vi "Config.Simulate.Set.vi"(8 "error in (no error)":errorcluster, 9 "Simulate":bool, 11 "Config Folder":path=path "C:/DDCS/Config") -> (0 "error out":errorcluster)   [LabVIEW 2024, in "EQMF.lvlib" / "Config Utils.lvlib"]
doc: "This VI writes the simulate flag (Boolean) to the station config INI file (Local Station.ini).\nThe Simulate flag is stored in section \"Simulate\" item \"Enable\".\n\nINPUTS:\n<B>Config folder</B> - This is the folder where config files are stored.\n<B>Simulate</B> - This is the state to be stored. TRUE equals Simulate is ON.\n\nOUTPUTS:\nNone\n\nERRORS: \nIf the config file cannot be created or written to, an error will be reported."
uses:
  Config Utils.lvlib
  <vilib>/Utility/config.llb/Write Key (Boolean).vi
  <vilib>/Utility/config.llb/NI_LVConfig.lvlib
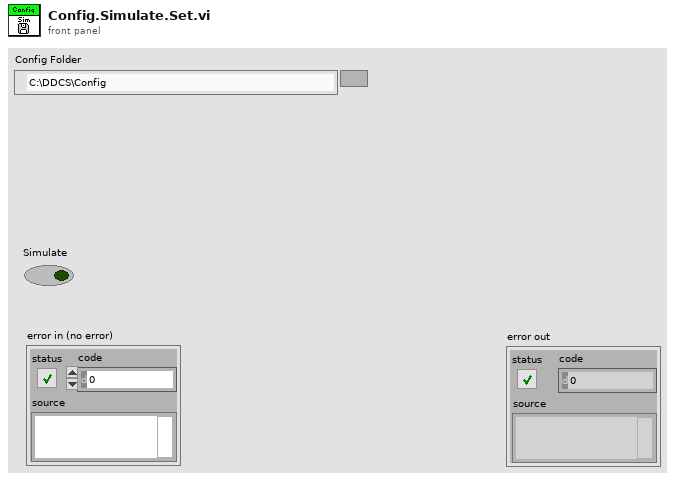
[diagram p1: front panel]
types:
  T1 = typedef "NI_LVConfig.lvlib/Config Data RefNum.ctl" = refnum<k1>
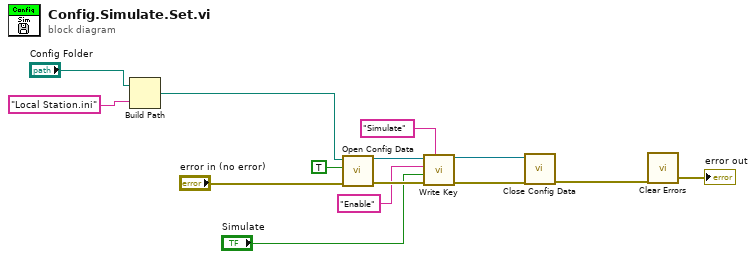
[diagram p0: block diagram]
diagram:
  n1 = Build Path(base path="Config Folder", name or relative path="Local Station.ini") -> (appended path=w12:path)
  n2 = call <vilib>:"Open Config Data.vi"("error in (no error)"="error in (no error)", "create file if necessary (T)"=TRUE, "configuration file path"=w12) -> ("error out"=w9:errorcluster, "refnum"=w10:T1)  [unwired: 6 in, 1 out]
  n3 = call-poly <vilib>:"Write Key.vi"("section"="Simulate", "error in (no error)"=w9, "value"="Simulate", "key"="Enable", "refnum"=w10) -> ("error out"=w5:errorcluster, "refnum out"=w6:T1)  [unwired: 4 in, 1 out]
  n4 = call <vilib>:"Close Config Data.vi"("error in (no error)"=w5, "refnum"=w6) -> ("error out"=w13:errorcluster)  [unwired: 8 in, 1 out]
  n5 = call <vilib>:"Clear Errors.vi"("error in (no error)"=w13) -> ("error out"=→"error out":errorcluster)  [unwired: 5 in, 1 out]
